vi "sendOutputData.vi"(8 "error in (no error)":errorcluster, 9 "outputData":T1 {"Step & Direction" min=-32767}, 10 "model":refnum<class "Model.lvclass">, 11 "State in":refnum<class "State.lvclass">) -> (0 "error out":errorcluster, 2 "model 2":refnum<class "Model.lvclass">, 3 "State out":refnum<class "State.lvclass">)   [LabVIEW 2012, in "State.lvclass"]
uses:
  State.lvclass
  Model/Model/Model.lvclass
  Program Files (x86)/National Instruments/LabVIEW 2012/user.lib/Common/ILC/Typedefs/OutputData.ctl
panel:
  # "DAC"
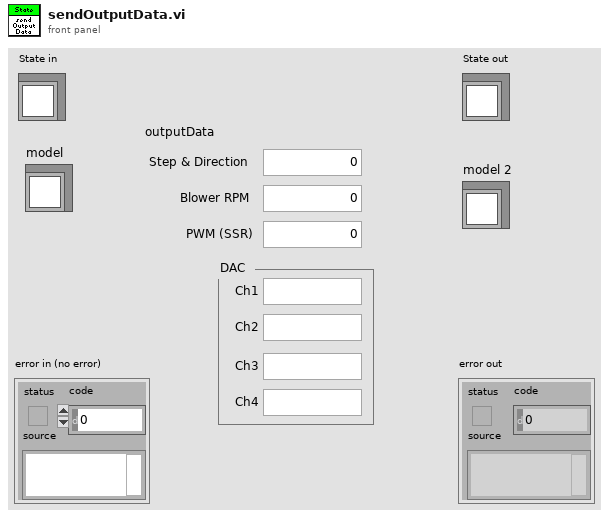
[diagram p1: front panel]
types:
  T1 = typedef "OutputData.ctl" = cluster{"Step & Direction":i16, "Blower RPM":u8, "PWM (SSR)":u8, "Ch1":u16, "Ch2":u16, "Ch3":u16, "Ch4":u16}
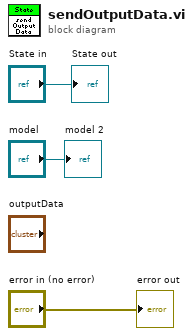
[diagram p0: block diagram]
diagram:
  "error out" <- "error in (no error)"
  "State out" <- "State in"
  "model 2" <- "model"
